vi "Translate Wheel_Ackermann.vi"(8 "error in (no error)":errorcluster, 9 "new position":cluster{"x":dbl, "y":dbl}, 10 "wheel index":i32, 11 "ackermann steering frame in":refnum<class "NI_Robotics_Ackermann Steering Frame.lvclass">) -> (0 "error out":errorcluster, 3 "ackermann steering frame out":refnum<class "NI_Robotics_Ackermann Steering Frame.lvclass">)   [LabVIEW 2017, in "NI_Robotics_Configure Steering Frame.lvlib"]
uses:
  <vilib>/robotics/Dialog/Configure Steering Frame/NI_Robotics_Configure Steering Frame.lvlib
  <vilib>/robotics/Steering/Ackermann Steering Frame/NI_Robotics_Ackermann Steering Frame.lvclass
  c:/Program Files (x86)/National Instruments/LabVIEW 2017/vi.lib/robotics/Steering/Steering Frame/NI_Robotics_Steering Frame.lvclass
  <vilib>/robotics/Steering/Ackermann Steering Frame/NI_Robotics_Ackermann Steering Frame.lvclass/NI_Robotics_Ackermann Steering Frame.ctl
  <vilib>/robotics/Steering/Steering Frame/NI_Robotics_Steering Frame.lvclass/NI_Robotics_Steering Frame.ctl
  <vilib>/robotics/Steering/Wheel/NI_Robotics_Wheel.lvclass/NI_Robotics_Wheel.ctl
  <vilib>/robotics/Steering/Ackermann Steering Frame/Wheel Separation to Frame Positions.vi
  <vilib>/robotics/Steering/Steering Frame/Reposition Wheels.vi
  <vilib>/robotics/Steering/Wheel/Update Steering to Wheel Frame Transform.vi
  <vilib>/Analysis/coordinate.llb/Wrap Angle.vi
  <vilib>/Analysis/coordinate.llb/Wrap Angle (scalar).vi
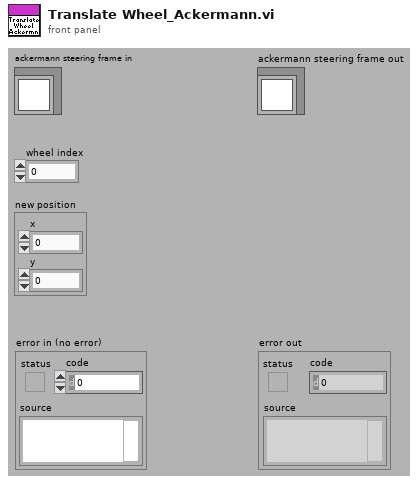
[diagram p1: front panel]
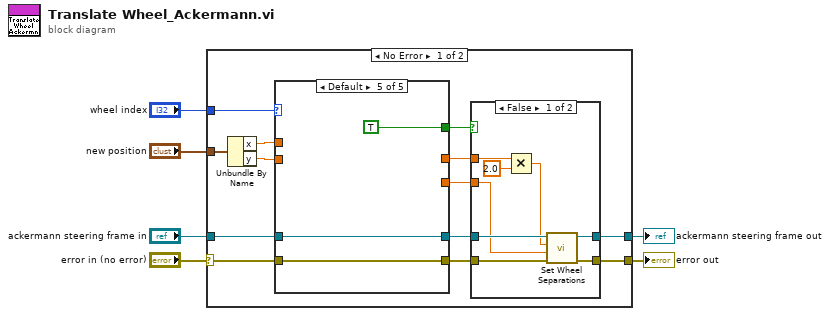
[diagram p0: block diagram]
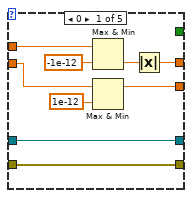
[diagram p3: hidden frame]
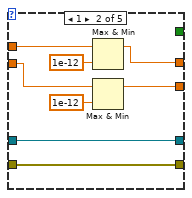
[diagram p4: hidden frame]
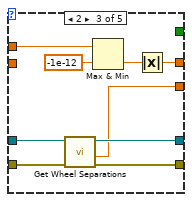
[diagram p5: hidden frame]
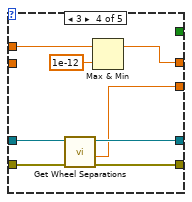
[diagram p6: hidden frame]
diagram:
  n1 = case shown="No Error" "error in (no error)" {
    selector: "error in (no error)" -> [w10 w67]
    tunnel: "ackermann steering frame in" -> [w9 w68]
    tunnel: [w15 w68] -> w4
    tunnel: [w14 w67] -> w3
    tunnel: "wheel index" -> [w19 _]
    tunnel: "new position" -> [w18 _]
    frame No Error {
      n2 = Unbundle By Name(w18) -> ("x"=w17:dbl, "y"=w16:dbl)
      n3 = case shown="Default" w19 {
        tunnel: w17 -> [w38 w46 w55 w63 _]
        tunnel: [w35 w45 w53 w56 _] -> w12
        tunnel: [_ _ _ _ TRUE] -> w13
        tunnel: w16 -> [w34 w42 _ _ _]
        tunnel: [w32 w41 w47 w57 _] -> w11
        tunnel: w10 -> [w30 w39 w50 w60 w64]
        tunnel: w9 -> [w31 w40 w51 w61 w65]
        tunnel: [w31 w40 w49 w59 w65] -> w8
        tunnel: [w30 w39 w48 w58 w64] -> w7
        frame 0 {
          n4 = Max & Min(x=w38, y=-1e-12) -> (min(x,y)=w36:dbl)  [unwired: 1 out]
          n5 = Max & Min(x=w34, y=1e-12) -> (max(x,y)=w32:dbl)  [unwired: 1 out]
          n6 = Absolute Value(x=w36) -> (abs(x)=w35:dbl)
        }
        frame 1 {
          n7 = Max & Min(x=w46, y=1e-12) -> (max(x,y)=w45:dbl)  [unwired: 1 out]
          n8 = Max & Min(x=w42, y=1e-12) -> (max(x,y)=w41:dbl)  [unwired: 1 out]
        }
        frame 2 {
          n9 = call <vilib>:"Get Wheel Separations.vi"("error in (no error)"=w50, "ackermann steering frame in"=w51) -> ("error out"=w48:errorcluster, "wheel separation length"=w47:dbl, "ackermann steering frame out"=w49:refnum<class "NI_Robotics_Ackermann Steering Frame.lvclass">)  [unwired: 6 in, 1 out]
          n10 = Max & Min(x=w55, y=-1e-12) -> (min(x,y)=w52:dbl)  [unwired: 1 out]
          n11 = Absolute Value(x=w52) -> (abs(x)=w53:dbl)
        }
        frame 3 {
          n12 = call <vilib>:"Get Wheel Separations.vi"("error in (no error)"=w60, "ackermann steering frame in"=w61) -> ("error out"=w58:errorcluster, "wheel separation length"=w57:dbl, "ackermann steering frame out"=w59:refnum<class "NI_Robotics_Ackermann Steering Frame.lvclass">)  [unwired: 6 in, 1 out]
          n13 = Max & Min(x=w63, y=1e-12) -> (max(x,y)=w56:dbl)  [unwired: 1 out]
        }
        frame Default {
        }
      }
      n14 = case shown="False" w13 {
        tunnel: w7 -> [w26 w28]
        tunnel: w8 -> [w27 w29]
        tunnel: [w25 w29] -> w15
        tunnel: [w24 w28] -> w14
        tunnel: w12 -> [w23 _]
        tunnel: w11 -> [w20 _]
        frame False {
          n15 = Multiply(x=w23, y=2.0) -> (x*y=w21:dbl)
          n16 = call <vilib>:"Set Wheel Separations.vi"("error in (no error)"=w26, "wheel separation length"=w20, "wheel separation width"=w21, "ackermann steering frame in"=w27) -> ("error out"=w24:errorcluster, "ackermann steering frame out"=w25:refnum<class "NI_Robotics_Ackermann Steering Frame.lvclass">)  [unwired: 6 in]
        }
        frame True {
        }
      }
    }
    frame Error {
    }
  }
  "ackermann steering frame out" <- w4
  "error out" <- w3
